vi "svx_DAQ_SetDefaults.vi"(7 "Channel Information In":T1={"Initialized?"=FALSE, "DAQmx Channel"="", "Channel Type"=0, "Max"=5.0, "Sensitivity"=1000.0, "Excitation"=FALSE, "Coupling"=enum."DC", "Location"="", "Orientation"="", "excitation"=enum."Off"} {"Max" min=0.0 format="± %^#_4g"; "Channel Type" items=["Voltage (V)"=0, "Charge (C)"=9, "-"=99, "SPL (Pa)"=3, "Force (lbf)"=6, "Force (N)"=1, "Acceleration (g) - IEPE"=2, "Acceleration (g) - Charge"=12, "Acceleration (g) - 4 wire DC Voltage"=22, "Velocity (in/s)"=7, "Velocity (mm/s)"=8, "Prox Probe (mil)"=4, "Prox Probe (mm)"=5]}) -> (8 "Channel Information Out":T1={"Initialized?"=FALSE, "DAQmx Channel"="", "Channel Type"=0, "Max"=5.0, "Sensitivity"=1000.0, "Excitation"=FALSE, "Coupling"=enum."DC", "Location"="", "Orientation"="", "excitation"=enum."Off"} {"Max" min=0.0 format="± %^#_4g"; "Channel Type" items=["Voltage (V)"=0, "Charge (C)"=9, "-"=99, "SPL (Pa)"=3, "Force (lbf)"=6, "Force (N)"=1, "Acceleration (g) - IEPE"=2, "Acceleration (g) - Charge"=12, "Acceleration (g) - 4 wire DC Voltage"=22, "Velocity (in/s)"=7, "Velocity (mm/s)"=8, "Prox Probe (mil)"=4, "Prox Probe (mm)"=5]})   [LabVIEW 2017, in "SVX NI-DAQmx AI Configuration XControl.xctl"]
uses:
  <vilib>/addons/Sound and Vibration/svt_DAQmx/Configuration XControl/SVX NI-DAQmx AI Configuration XControl.xctl
  <vilib>/addons/Sound and Vibration/svt_DAQmx/Configuration XControl/Controls/svx_DAQ_ChannelInfo.ctl
  <vilib>/addons/Sound and Vibration/svt_DAQmx/Configuration XControl/Controls/svx_DAQ_ChannelType.ctl
  <vilib>/addons/Sound and Vibration/svt_DAQmx/Configuration XControl/Controls/svx_DAQ_Coupling.ctl
  <vilib>/addons/Sound and Vibration/svt_DAQmx/Configuration XControl/Controls/svx_DAQ_Excitation.ctl
  <resource>/objmgr/daqmx.rc
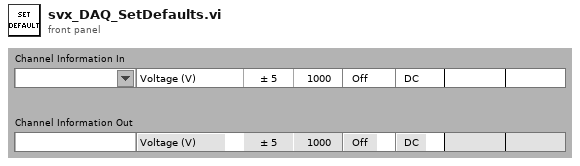
[diagram p1: front panel]
types:
  T1 = typedef "SVX NI-DAQmx AI Configuration XControl.xctl/svx_DAQ_ChannelInfo.ctl" = cluster{"Initialized?":bool, "DAQmx Channel":tag, "Channel Type":T2, "Max":dbl, "Sensitivity":dbl, "Excitation":bool, "Coupling":T3, "Location":string, "Orientation":string, "excitation":T4}
  T2 = typedef "SVX NI-DAQmx AI Configuration XControl.xctl/svx_DAQ_ChannelType.ctl" = u16
  T3 = typedef "SVX NI-DAQmx AI Configuration XControl.xctl/svx_DAQ_Coupling.ctl" = enum16{"AC", "DC"}
  T4 = typedef "svx_DAQ_Excitation.ctl" = enum16{"Off", "Min", "Max"}
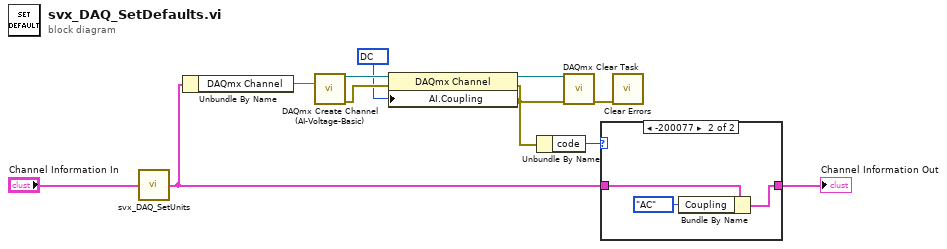
[diagram p0: block diagram]
diagram:
  w8 = 10050 items=["AC"=10045, "DC"=10050, "GND"=10066] ("AI.Coupling")
  n1 = call <vilib>:"svx_DAQ_SetUnits.vi"("Channel Information In"="Channel Information In") -> ("Channel Information Out"=w3:T1)  [unwired: 4 in]
  n2 = Unbundle By Name(w3) -> ("DAQmx Channel"=w11:tag)
  n3 = call <vilib>:"DAQmx Create Channel (AI-Voltage-Basic).vi"("physical channels"=w11) -> ("task out"=w10:refnum<k21>, "error out"=w9:errorcluster)  [unwired: 13 in]
  n4 = property class="DAQmx Channel"(reference=w10, error in=w9, "AI.Coupling"=w8) -> (reference out=w5:refnum<k21>, error out=w6:errorcluster)
  n5 = Unbundle By Name(w6) -> ("code"=w7:i32)
  n6 = call <vilib>:"DAQmx Clear Task.vi"("task in"=w5, "error in"=w6) -> ("error out"=w4:errorcluster)  [unwired: 13 in]
  n7 = case shown="-200077" w7 {
    tunnel: w3 -> [w12 w15]
    tunnel: [w12 w13] -> w1
    frame Default {
    }
    frame -200077 {
      n8 = Bundle By Name(cluster=w15, "Coupling"=svx_DAQ_Coupling."AC") -> (w13:T1)
    }
  }
  "Channel Information Out" <- w1
  n9 = call <vilib>:"Clear Errors.vi"("error in (no error)"=w4) -> ()  [unwired: 5 in, 2 out]
